vi "Is stopped.vi"(8 "error in (no error)":errorcluster, 11 "Mag Lab Root in":refnum<class "Mag Lab Root.lvclass">) -> (0 "error out":errorcluster, 2 "Boolean":bool, 3 "Mag Lab Root out":refnum<class "Mag Lab Root.lvclass">)   [LabVIEW 2015, in "Mag Lab Root.lvclass"]
uses:
  Mag Lab Root.lvclass
  Mag Lab Root.lvclass/Mag Lab Root.ctl
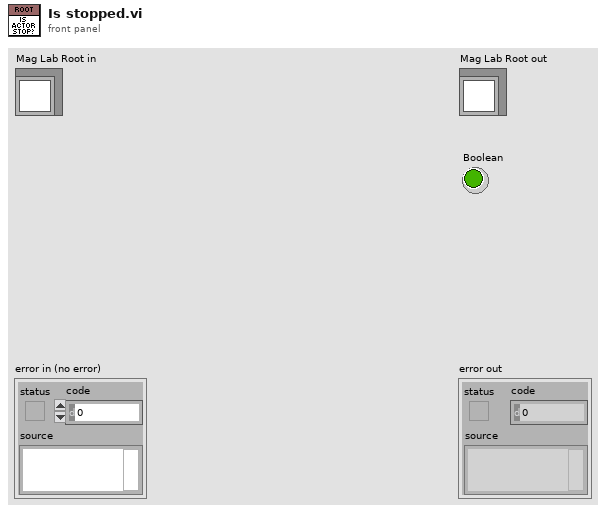
[diagram p1: front panel]
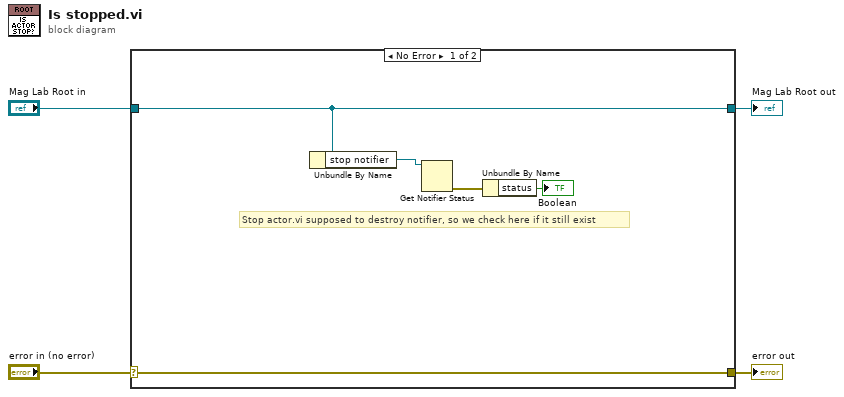
[diagram p0: block diagram]
diagram:
  n1 = case shown="No Error" "error in (no error)" {
    selector: "error in (no error)" -> [w9 w11]
    tunnel: [w9 w11] -> w3
    tunnel: [w8 w10] -> w1
    tunnel: "Mag Lab Root in" -> [w8 w10]
    frame No Error {
      # "Stop actor.vi supposed to destroy notifier, so we check here if it still exist"
      n2 = Unbundle By Name(w8) -> ("stop notifier"=w7:refnum<notifier>)
      n3 = Get Notifier Status(notifier=w7) -> (error out=w6:errorcluster)  [unwired: 1 in, 4 out]
      n4 = Unbundle By Name(w6) -> ("status"=→"Boolean":bool)
    }
    frame Error {
    }
  }
  "error out" <- w3
  "Mag Lab Root out" <- w1
